vi "Overlay Results (CoordSys Pattern).vi"(4 "Match":T4 {"Bounding Box"."y" format="%.2f"; "Bounding Box"."x" format="%.2f"; "Position"."y" format="%.2f"; "Position"."x" format="%.2f"; "Score" format="%.2f"; "Scale" format="%.2f"; "Angle" format="%.2f"}, 6 "Axis 2":T1 {"Point 2"."Y" format="%.2f"; "Point 2"."X" format="%.2f"; "Point 1"."Y" format="%.2f"; "Point 1"."X" format="%.2f"}, 7 "Setup":T3, 8 "error in (no error)":errorcluster, 9 "Axis 1":T1 {"Point 2"."Y" format="%.2f"; "Point 2"."X" format="%.2f"; "Point 1"."Y" format="%.2f"; "Point 1"."X" format="%.2f"}, 10 "Search Rect":T2 {"Rotation" min=-90.0 max=90.0 step=1.0 format="%.2f"; "Left" scale=0.0..1024.0; "Right" scale=0.0..1024.0}, 11 "Image In":T5) -> (0 "error out":errorcluster, 3 "Image Out":T5)   [LabVIEW 2016]
uses:
  <vilib>/vision/Image Controls.llb/IMAQ Image.ctl
panel:
  in  "Feature Found Color":u32(colorbox)=16776960
  in  "Result Color":u32(colorbox)=16711680
  in  "Search Area Color":u32(colorbox)=65280
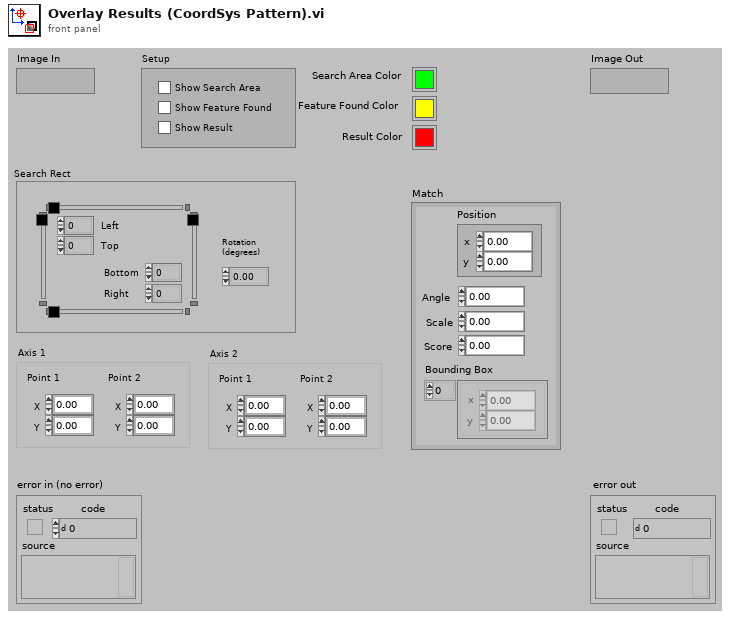
[diagram p1: front panel]
types:
  T1 = cluster{"Point 1":cluster{"X":sgl, "Y":sgl}, "Point 2":cluster{"X":sgl, "Y":sgl}}
  T2 = typedef "IMAQ Rectangle" = cluster{"Left":i32, "Top":i32, "Right":i32, "Bottom":i32, "Rotation":dbl}
  T3 = cluster{"Show Search Area":bool, "Show Feature Found":bool, "Show Result":bool}
  T4 = cluster{"Position":cluster{"x":sgl, "y":sgl}, "Angle":sgl, "Scale":sgl, "Score":sgl, "Bounding Box":cluster{"x":sgl, "y":sgl}[]}
  T5 = typedef "IMAQ Image.ctl" = refnum<image>
  T6 = cluster{"Left":i32, "Top":i32, "Right":i32, "Bottom":i32}
  T7 = cluster{"[0]":sgl, "[1]":sgl, "[2]":sgl, "[3]":sgl}
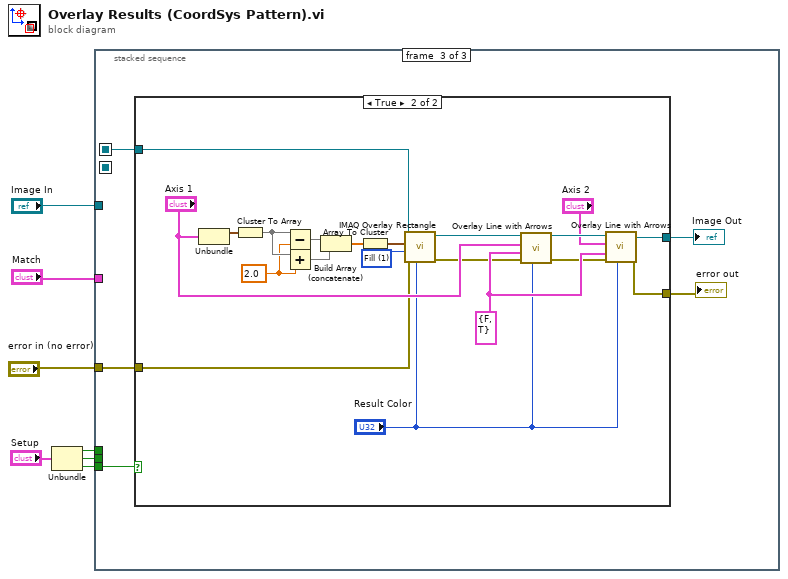
[diagram p0: block diagram]
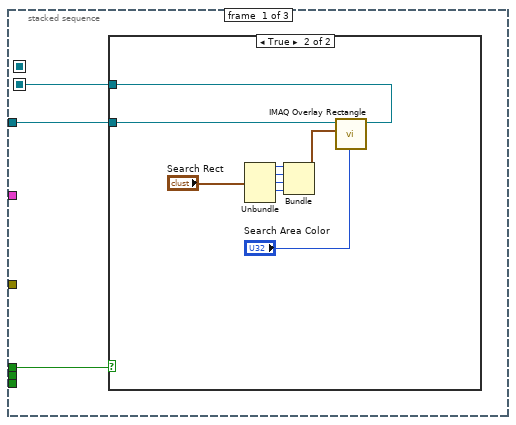
[diagram p2: hidden frame]
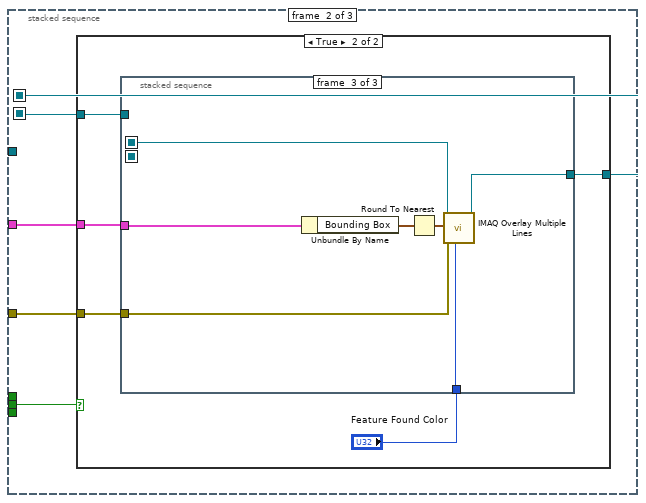
[diagram p4: hidden frame]
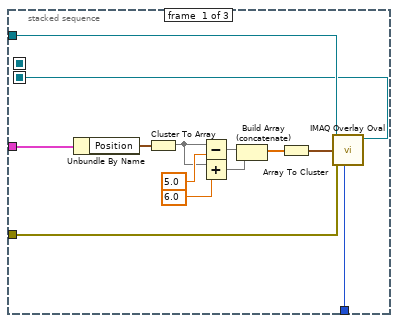
[diagram p6: hidden frame]
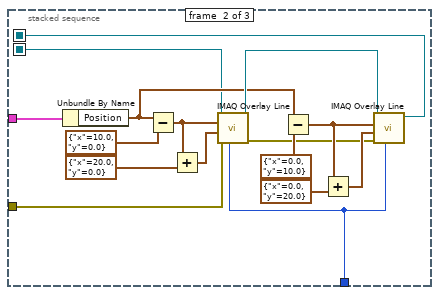
[diagram p7: hidden frame]
diagram:
  n1 = Unbundle("Setup") -> ("Show Search Area"=w3:bool, "Show Feature Found"=w4:bool, "Show Result"=w2:bool)
  n2 = stacked-sequence {
    seq-local: [w8 _ _] -> [_ w23 _]
    seq-local: [_ w22 _] -> [_ _ w71]
    tunnel: "Image In" -> [w9 _ _]
    tunnel: "Match" -> [_ w24 _]
    tunnel: w4 -> [_ w25 _]
    tunnel: w3 -> [w10 _ _]
    tunnel: w2 -> [_ _ w72]
    tunnel: "error in (no error)" -> [_ w21 w68]
    frame #0 {
      n3 = case shown="True" w10 {
        tunnel: w9 -> [w11 w20]
        tunnel: [w11 w13] -> w8
        frame False {
        }
        frame True {
          n4 = Unbundle("Search Rect") -> ("Left"=w18:i32, "Top"=w17:i32, "Right"=w16:i32, "Bottom"=w15:i32)  [unwired: 1 out]
          n5 = Bundle("Left"=w18, "Top"=w17, "Right"=w16, "Bottom"=w15) -> (w12:T6)  [unwired: 1 out]
          n6 = call "IMAQ Overlay Rectangle"("Color"="Search Area Color", "Rectangle"=w12, "Image"=w20) -> ("Image Out"=w13:T5)  [unwired: 3 in, 5 out]
        }
      }
    }
    frame #1 {
      n7 = case shown="True" w25 {
        tunnel: [w26 w30] -> w22
        tunnel: w24 -> [_ w31]
        tunnel: w23 -> [w26 w29]
        tunnel: w21 -> [_ w28]
        frame False {
        }
        frame True {
          n8 = stacked-sequence {
            seq-local: [w37 _ _] -> [_ w49 _]
            seq-local: [_ w48 _] -> [_ _ w66]
            tunnel: w31 -> [w36 w50 w67]
            tunnel: w29 -> [w38 _ _]
            tunnel: [_ _ w64] -> w30
            tunnel: w28 -> [w33 w45 w61]
            tunnel: "Feature Found Color" -> [w32 w46 w62]
            frame #0 {
              n9 = Unbundle By Name(w36) -> ("Position"=w35:cluster{"x":sgl, "y":sgl})
              n10 = Cluster To Array(cluster=w35) -> (array=w40:sgl[])
              n11 = Subtract(x=w40, y=sgl 5.0) -> (x-y=w44:sgl[])
              n12 = Add(x=w40, y=sgl 6.0) -> (x+y=w43:sgl[])
              n13 = Build Array (concatenate)(w44, w43) -> (w39:sgl[])
              n14 = Array To Cluster(array=w39) -> (cluster=w34:T7)
              n15 = call "IMAQ Overlay Oval"("Color"=w32, "error in (no error)"=w33, "Bounding Rectangle"=w34, "Image"=w38) -> ("Image Out"=w37:T5)  [unwired: 2 in, 5 out]
            }
            frame #1 {
              n16 = Unbundle By Name(w50) -> ("Position"=w51:cluster{"x":sgl, "y":sgl})
              n17 = Subtract(x=w51, y=cluster{"x":sgl, "y":sgl} {"x"=10.0, "y"=0.0}) -> (x-y=w57:cluster{"x":sgl, "y":sgl})
              n18 = Add(x=w57, y=cluster{"x":sgl, "y":sgl} {"x"=20.0, "y"=0.0}) -> (x+y=w58:cluster{"x":sgl, "y":sgl})
              n19 = call "IMAQ Overlay Line"("Color"=w46, "error in (no error)"=w45, "End Point"=w58, "Start Point"=w57, "Image"=w49) -> ("error out"=w47:errorcluster, "Image Out"=w52:T5)  [unwired: 1 in, 4 out]
              n20 = Subtract(x=w51, y=cluster{"x":sgl, "y":sgl} {"x"=0.0, "y"=10.0}) -> (x-y=w56:cluster{"x":sgl, "y":sgl})
              n21 = Add(x=w56, y=cluster{"x":sgl, "y":sgl} {"x"=0.0, "y"=20.0}) -> (x+y=w55:cluster{"x":sgl, "y":sgl})
              n22 = call "IMAQ Overlay Line"("Color"=w46, "error in (no error)"=w47, "End Point"=w55, "Start Point"=w56, "Image"=w52) -> ("Image Out"=w48:T5)  [unwired: 1 in, 5 out]
            }
            frame #2 {
              n23 = Unbundle By Name(w67) -> ("Bounding Box"=w65:cluster{"x":sgl, "y":sgl}[])
              n24 = Round To Nearest(number=w65) -> (nearest integer value=w63:cluster{"x":sgl, "y":sgl}[])
              n25 = call "IMAQ Overlay Multiple Lines"("Color"=w62, "error in (no error)"=w61, "Line End Points"=w63, "Image"=w66) -> ("Image Out"=w64:T5)  [unwired: 2 in, 5 out]
            }
          }
        }
      }
    }
    frame #2 {
      n26 = case shown="True" w72 {
        tunnel: [w74 w92] -> w70
        tunnel: w71 -> [w74 w81]
        tunnel: [w73 w76] -> w69
        tunnel: w68 -> [w73 w75]
        frame False {
        }
        frame True {
          w79 = u32 1 items=["Frame", "Fill", "Highlight"] ("Drawing Mode (Frame)")
          w84 = sgl 2.0
          w93 = cluster{"Start point":bool, "End point":bool} {"Start point"=FALSE, "End point"=TRUE} ("Arrows")
          n27 = Unbundle("Axis 1") -> ("Point 1"=w90:cluster{"X":sgl, "Y":sgl})  [unwired: 1 out]
          n28 = Cluster To Array(cluster=w90) -> (array=w86:sgl[])
          n29 = Subtract(x=w86, y=w84) -> (x-y=w89:sgl[])
          n30 = Add(x=w86, y=w84) -> (x+y=w85:sgl[])
          n31 = Build Array (concatenate)(w89, w85) -> (w88:sgl[])
          n32 = Array To Cluster(array=w88) -> (cluster=w87:T7)
          n33 = call "IMAQ Overlay Rectangle"("Color"="Result Color", "error in (no error)"=w75, "Drawing Mode (Frame)"=w79, "Rectangle"=w87, "Image"=w81) -> ("error out"=w78:errorcluster, "Image Out"=w80:T5)  [unwired: 1 in, 4 out]
          n34 = call <vilib>:"Overlay Line with Arrows.vi"("Color"="Result Color", "error in (no error)"=w78, "Arrows"=w93, "Line Coordinates"="Axis 1", "Image In"=w80) -> ("error out"=w77:errorcluster, "Image Out"=w94:T5)  [unwired: 1 in, 4 out]
          n35 = call <vilib>:"Overlay Line with Arrows.vi"("Color"="Result Color", "error in (no error)"=w77, "Arrows"=w93, "Line Coordinates"="Axis 2", "Image In"=w94) -> ("error out"=w76:errorcluster, "Image Out"=w92:T5)  [unwired: 1 in, 4 out]
        }
      }
      "Image Out" <- w70
      "error out" <- w69
    }
  }
